vi "Close DSI.vi"(8 "error in":errorcluster, 11 "DSI Reference":refnum<class "DCM-DSI.lvclass">) -> (0 "error out":errorcluster)   [LabVIEW 2016, in "DCM-DSI.lvclass"]
uses:
  DCM-DSI.lvclass
  DCM-DSI.lvclass/DCM-DSI.ctl
  <vilib>/Powertrain Controls/Device Drivers/DCM/Rev0/RT/DCM - RT.lvclass/DCM - RT.ctl
  <vilib>/Powertrain Controls/Device Drivers/DCM/Rev0/RT/Write Stop Target.vi
  <vilib>/Powertrain Controls/Device Drivers/DCM/Rev0/RT/DCM - RT.lvclass
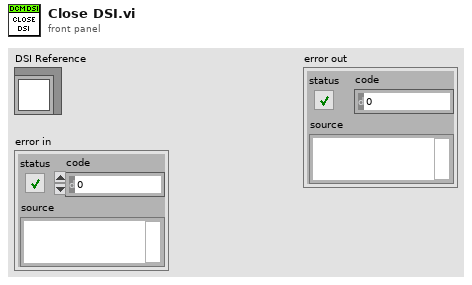
[diagram p1: front panel]
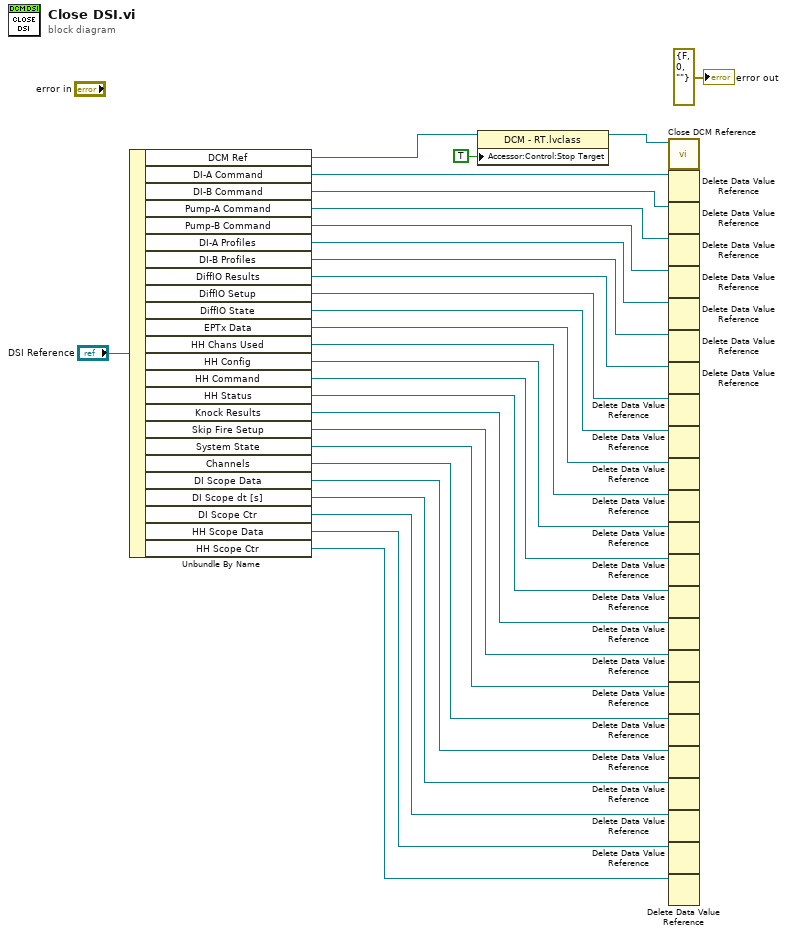
[diagram p0: block diagram]
diagram:
  n1 = Unbundle By Name("DSI Reference") -> ("DCM Ref"=w3:refnum<class "DCM - RT.lvclass">, "DI-A Command"=w27:refnum<data-value>, "DI-B Command"=w26:refnum<data-value>, "Pump-A Command"=w25:refnum<data-value>, "Pump-B Command"=w24:refnum<data-value>, "DI-A Profiles"=w23:refnum<data-value>, "DI-B Profiles"=w22:refnum<data-value>, "DiffIO Results"=w21:refnum<data-value>, "DiffIO Setup"=w20:refnum<data-value>, "DiffIO State"=w19:refnum<data-value>, "EPTx Data"=w11:refnum<data-value>, "HH Chans Used"=w18:refnum<data-value>, "HH Config"=w17:refnum<data-value>, "HH Command"=w16:refnum<data-value>, "HH Status"=w15:refnum<data-value>, "Knock Results"=w10:refnum<data-value>, "Skip Fire Setup"=w14:refnum<data-value>, "System State"=w13:refnum<data-value>, "Channels"=w12:refnum<data-value>, "DI Scope Data"=w8:refnum<data-value>, "DI Scope dt [s]"=w7:refnum<data-value>, "DI Scope Ctr"=w6:refnum<data-value>, "HH Scope Data"=w5:refnum<data-value>, "HH Scope Ctr"=w4:refnum<data-value>)
  n2 = property class="DCM - RT.lvclass"(reference=w3, "Accessor:Control:Stop Target"=TRUE ("Stop Target")) -> (reference out=w1:refnum<class "DCM - RT.lvclass">)  [unwired: 1 in, 1 out]
  n3 = call <vilib>:"Close DCM Reference.vi"("DCM - RT in"=w1) -> ()  [unwired: 11 in]
  n4 = Delete Data Value Reference(data value reference=w27) -> ()  [unwired: 1 in, 2 out]
  n5 = Delete Data Value Reference(data value reference=w26) -> ()  [unwired: 1 in, 2 out]
  n6 = Delete Data Value Reference(data value reference=w25) -> ()  [unwired: 1 in, 2 out]
  n7 = Delete Data Value Reference(data value reference=w24) -> ()  [unwired: 1 in, 2 out]
  n8 = Delete Data Value Reference(data value reference=w23) -> ()  [unwired: 1 in, 2 out]
  n9 = Delete Data Value Reference(data value reference=w22) -> ()  [unwired: 1 in, 2 out]
  n10 = Delete Data Value Reference(data value reference=w21) -> ()  [unwired: 1 in, 2 out]
  n11 = Delete Data Value Reference(data value reference=w20) -> ()  [unwired: 1 in, 2 out]
  n12 = Delete Data Value Reference(data value reference=w19) -> ()  [unwired: 1 in, 2 out]
  n13 = Delete Data Value Reference(data value reference=w11) -> ()  [unwired: 1 in, 2 out]
  n14 = Delete Data Value Reference(data value reference=w18) -> ()  [unwired: 1 in, 2 out]
  n15 = Delete Data Value Reference(data value reference=w17) -> ()  [unwired: 1 in, 2 out]
  n16 = Delete Data Value Reference(data value reference=w16) -> ()  [unwired: 1 in, 2 out]
  n17 = Delete Data Value Reference(data value reference=w15) -> ()  [unwired: 1 in, 2 out]
  n18 = Delete Data Value Reference(data value reference=w10) -> ()  [unwired: 1 in, 2 out]
  n19 = Delete Data Value Reference(data value reference=w14) -> ()  [unwired: 1 in, 2 out]
  n20 = Delete Data Value Reference(data value reference=w13) -> ()  [unwired: 1 in, 2 out]
  n21 = Delete Data Value Reference(data value reference=w12) -> ()  [unwired: 1 in, 2 out]
  n22 = Delete Data Value Reference(data value reference=w8) -> ()  [unwired: 1 in, 2 out]
  n23 = Delete Data Value Reference(data value reference=w7) -> ()  [unwired: 1 in, 2 out]
  n24 = Delete Data Value Reference(data value reference=w6) -> ()  [unwired: 1 in, 2 out]
  n25 = Delete Data Value Reference(data value reference=w5) -> ()  [unwired: 1 in, 2 out]
  n26 = Delete Data Value Reference(data value reference=w4) -> ()  [unwired: 1 in, 2 out]
  "error out" <- errorcluster {"status"=FALSE, "code"=0, "source"=""} ("error out")
